vi "ADO Connection Create Parameterized Query.vi"(6 "stored procedure? (F)":bool, 7 "auto-detect parameters? (F)":bool, 8 "error in (no error)":errorcluster caption="错误输入（无错误）", 9 "parameters":T1[](array[typedef]), 10 "SQL query":string, 11 "Database Connection 输入":refnum<class "Database Connection.lvclass"> caption="DNL_LabVIEW Object in") -> (0 "error out":errorcluster caption="错误输出", 1 "parameters out":T1[](array[typedef]), 2 "Database Command 输出":refnum<class "Database Command.lvclass">, 3 "Database Connection 输出":refnum<class "Database Connection.lvclass"> caption="DNL_LabVIEW Object out")   [LabVIEW 2011, in "Database Connection.lvclass"]
uses:
  Database Connection.lvclass
  <vilib>/addons/database/Auxilliary.llb/DB Tools Parameter Info.ctl
  <vilib>/addons/database/Auxilliary.llb/DB Tools DataTypes.ctl
  <vilib>/addons/database/Auxilliary.llb/DB Tools Parameter Dir.ctl
  Command/Database Command.lvclass
  Database Connection.lvclass/Database Connection.ctl
  <vilib>/addons/database/NI_Database_API.lvlib
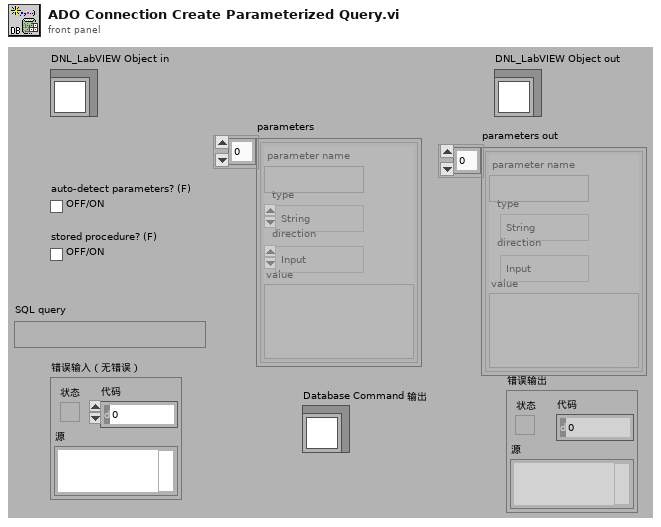
[diagram p1: front panel]
types:
  T1 = typedef "NI_Database_API.lvlib/DB Tools Parameter Info.ctl" = cluster{"parameter name":string, "type":T2, "direction":T3, "value":variant}
  T2 = typedef "NI_Database_API.lvlib/DB Tools DataTypes.ctl" = enum16{"String", "Long (I32)", "Single (SGL)", "Double (DBL)", "Date/Time", "Binary"}
  T3 = typedef "NI_Database_API.lvlib/DB Tools Parameter Dir.ctl" = enum32{"Input", "Output", "Input/Output", "Return Value"}
  T4 = cluster{"command timeout (s)":i32, "connection string":string, "default database":string, "provider":string}
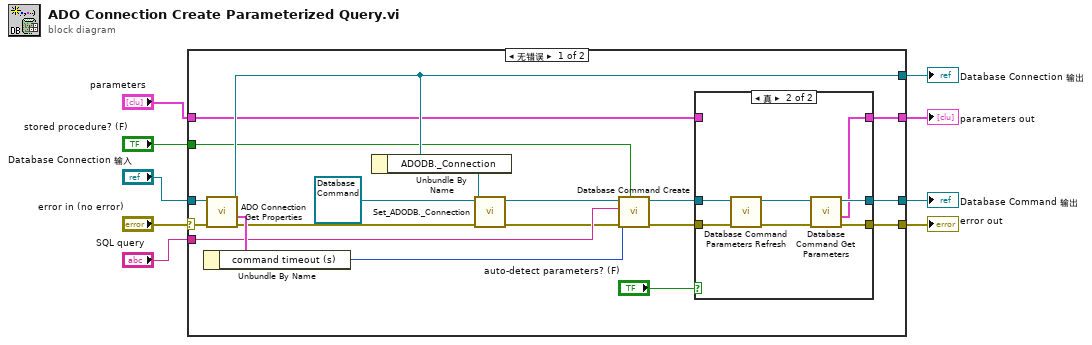
[diagram p0: block diagram]
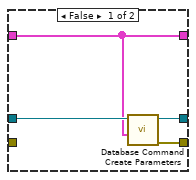
[diagram p2: hidden frame]
diagram:
  n1 = case shown="无错误" "error in (no error)" {
    selector: "error in (no error)" -> [w21 w40]
    tunnel: [w27 w41] -> w7
    tunnel: "Database Connection 输入" -> [w28 w41]
    tunnel: "SQL query" -> [w17 _]
    tunnel: "stored procedure? (F)" -> [w19 _]
    tunnel: "parameters" -> [w25 _]
    tunnel: [w24 _] -> w3
    tunnel: [w23 _] -> w2
    tunnel: [w22 w40] -> w1
    frame No Error {
      n2 = call "ADO Connection Get Properties.vi"("error in (no error)"=w21, "Database Connection 输入"=w28) -> ("error out"=w13:errorcluster, "connection properties"=w26:T4, "Database Connection 输出"=w27:refnum<class "Database Connection.lvclass">)  [unwired: 7 in]
      n3 = Unbundle By Name(w26) -> ("command timeout (s)"=w18:i32)
      n4 = Unbundle By Name(w27) -> ("ADODB._Connection"=w20:refnum<k7>)
      n5 = call "Set_ADODB._Connection.vi"("error in (no error)"=w13, "ADODB._Connection"=w20, "Database Command输入"=refnum<class "Database Command.lvclass"> refnum ("Database Command.lvclass")) -> ("error out"=w12:errorcluster, "Database Command输出"=w10:refnum<class "Database Command.lvclass">)  [unwired: 7 in]
      n6 = call "Database Command Create.vi"("stored procedure? (F)"=w19, "error in (no error)"=w12, "CommandTimeout"=w18, "SQL query"=w17, "Database Command 输入"=w10) -> ("error out"=w14:errorcluster, "Database Command 输出"=w15:refnum<class "Database Command.lvclass">)  [unwired: 5 in]
      n7 = case shown="真" "auto-detect parameters? (F)" {
        tunnel: w25 -> [w31 _]
        tunnel: [w31 w37] -> w24
        tunnel: [w30 w39] -> w23
        tunnel: [w29 w38] -> w22
        tunnel: w15 -> [w32 w36]
        tunnel: w14 -> [_ w33]
        frame False {
          n8 = call "Database Command Create Parameters.vi"("parameters"=w31, "Database Command 输入"=w32) -> ("error out"=w29:errorcluster, "Database Command 输出"=w30:refnum<class "Database Command.lvclass">)  [unwired: 8 in]
        }
        frame True {
          n9 = call "Database Command Parameters Refresh.vi"("error in (no error)"=w33, "Database Command 输入"=w36) -> ("error out"=w34:errorcluster, "Database Command 输出"=w35:refnum<class "Database Command.lvclass">)  [unwired: 8 in]
          n10 = call "Database Command Get Parameters.vi"("error in (no error)"=w34, "Database Command 输入"=w35) -> ("error out"=w38:errorcluster, "parameters"=w37:T1[], "Database Command 输出"=w39:refnum<class "Database Command.lvclass">)  [unwired: 7 in]
        }
      }
    }
    frame Error {
    }
  }
  "error out" <- w1
  "Database Connection 输出" <- w7
  "parameters out" <- w3
  "Database Command 输出" <- w2
